vi "消息推送core.vi"(8 "error in (no error)":errorcluster caption="错误输入（无错误）", 10 "数组":string[](array[string])=["UID_u2gUaG5SHjMBZfWcukaJD0Ypef0K"], 11 "content":string) -> (0 "error out":errorcluster caption="错误输出", 3 "GBK":string)   [LabVIEW 2016, in "wxpusher.lvlib"]
uses:
  wxpusher.lvlib
  <vilib>/httpClient/POSTBuffer.vi
  <vilib>/httpClient/LabVIEWHTTPClient.lvlib
panel:
  out "JSON字符串":string
  out "headers":string caption="头部"
  out "body":string caption="体部"
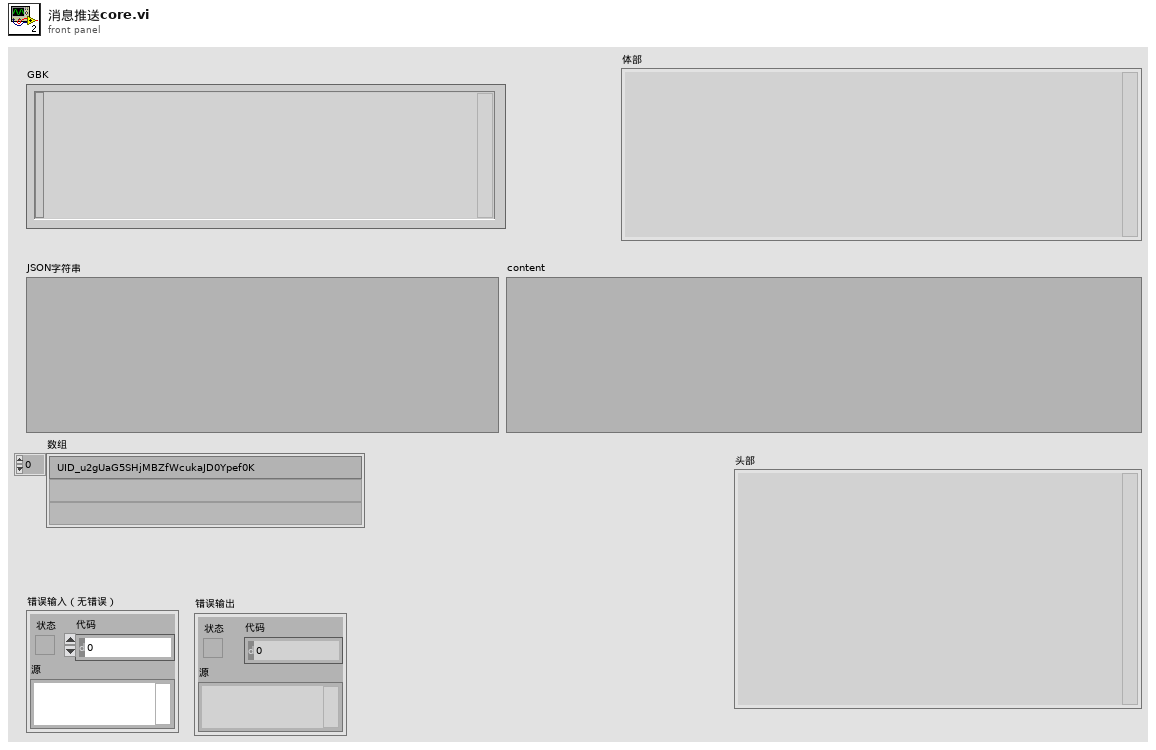
[diagram p1: front panel]
types:
  T1 = cluster{"appToken":string, "content":string, "contentType":i32, "topicIds":i32[], "uids":string[], "url":string}
  T2 = typedef "LabVIEWHTTPClient.lvlib/ClientHandle.ctl" = refnum<k1>
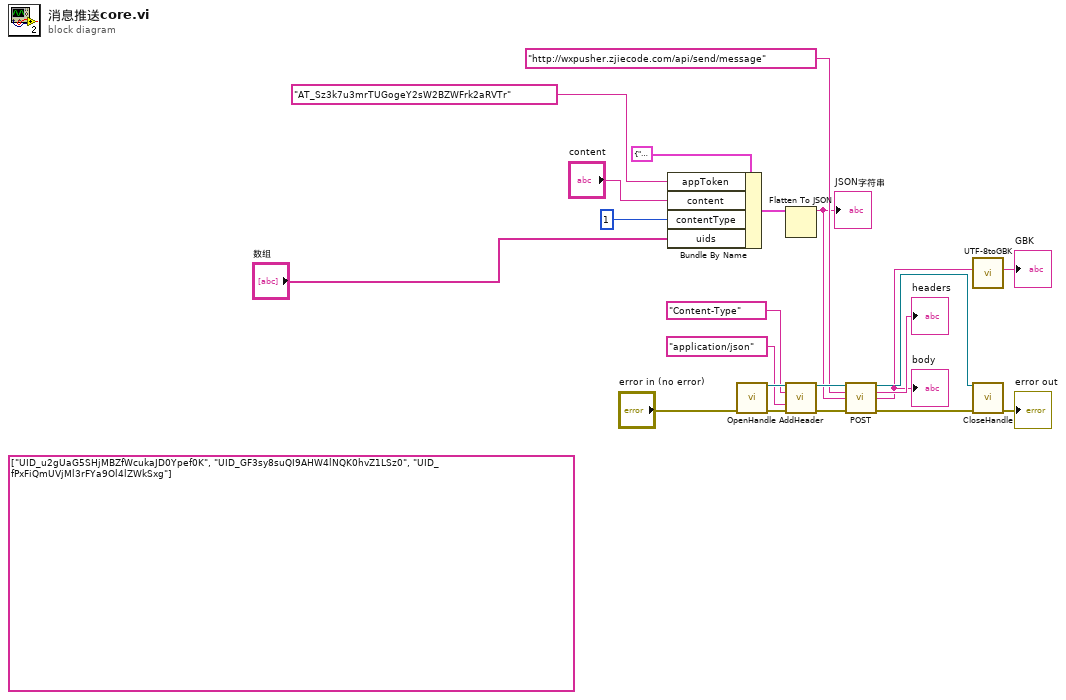
[diagram p0: block diagram]
diagram:
  (unwired) string[] ["UID_u2gUaG5SHjMBZfWcukaJD0Ypef0K", "UID_GF3sy8suQI9AHW4lNQK0hvZ1LSz0", "UID_fPxFiQmUVjMl3rFYa9Ol4lZWkSxg"]
  n1 = Bundle By Name(cluster=T1 {"appToken"="", "content"="", "contentType"=0, "topicIds"=[], "uids"=[], "url"=""}, "appToken"="AT_Sz3k7u3mrTUGogeY2sW2BZWFrk2aRVTr", "content"="content", "contentType"=1, "uids"="数组") -> (w8:T1)
  n2 = call <vilib>:"OpenHandle.vi"("error in (no error)"="error in (no error)") -> ("client handle out"=w21:T2, "error out"=w19:errorcluster)  [unwired: 13 in]
  n3 = Flatten To JSON(anything=w8) -> (JSON string=w7:string)  [unwired: 2 in, 1 out]
  "JSON字符串" <- w7
  n4 = call <vilib>:"AddHeader.vi"("client handle"=w21, "header"="Content-Type", "value"="application/json", "error in (no error)"=w19) -> ("client handle out"=w20:T2, "error out"=w16:errorcluster)  [unwired: 10 in]
  n5 = call-poly <vilib>:"POST.vi"("client handle"=w20, "url"="http://wxpusher.zjiecode.com/api/send/message", "buffer"=w7, "error in (no error)"=w16) -> ("client handle out"=w13:T2, "headers"=→"headers":string, "body"=w6:string, "error out"=w14:errorcluster)  [unwired: 8 in]
  "body" <- w6
  n6 = call "UTF-8toGBK.vi"("UTF-8"=w6) -> ("GBK"=→"GBK":string)  [unwired: 9 in, 1 out]
  n7 = call <vilib>:"CloseHandle.vi"("client handle"=w13, "error in (no error)"=w14) -> ("error out"=→"error out":errorcluster)  [unwired: 13 in]
